vi "dfd_Calculate FIR Transposed.vi"(4 "coef idx":T1={"start"=0, "stepsize"=1}, 5 "#taps per phase":i32, 6 "coef":i64[](array[numeric]), 7 "Fwldiff":i16, 9 "state idx":T1={"start"=0, "stepsize"=1}, 10 "state in":i64[](array[numeric]), 11 "x":i64) -> (2 "state out":i64[](array[numeric]))   [LabVIEW 2017, in "NI_DigFilter_FXP.lvlib"]
uses:
  <vilib>/addons/Digital Filter Design/NI_DigFilter_FXP.lvlib
  <vilib>/addons/Digital Filter Design/_Objects.llb/dfd_Index Config.ctl
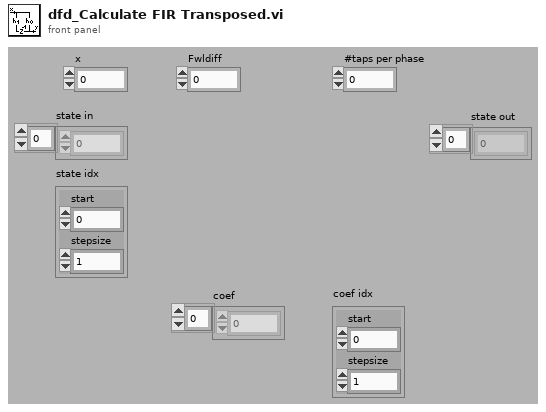
[diagram p1: front panel]
types:
  T1 = typedef "dfd_Index Config.ctl" = cluster{"start":i32, "stepsize":i32}
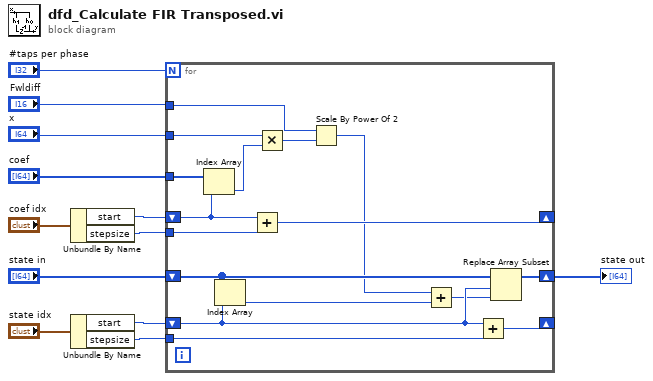
[diagram p0: block diagram]
diagram:
  n1 = Unbundle By Name("coef idx") -> ("start"=w12:i32, "stepsize"=w11:i32)
  n2 = Unbundle By Name("state idx") -> ("start"=w9:i32, "stepsize"=w10:i32)
  n3 = for {
    N: "#taps per phase" -> [_]
    shift-right: [w23] -> w2
    shift-left: "state in" -> [w24]
    shift-right: [w25] -> _
    shift-left: w12 -> [w27]
    tunnel: "coef" -> [w28]
    tunnel: w11 -> [w26]
    tunnel: "x" -> [w17]
    shift-right: [w20] -> _
    shift-left: w9 -> [w22]
    tunnel: w10 -> [w21]
    tunnel: "Fwldiff" -> [w13]
    n4 = Index Array(array=w28, index=w27) -> (element=w16:i64)
    n5 = Index Array(array=w24, index=w22) -> (element=w18:i64)
    n6 = Add(x=w27, y=w26) -> (x+y=w25:i32)
    n7 = Multiply(x=w17, y=w16) -> (x*y=w15:i64)
    n8 = Scale By Power Of 2(n=w13, x=w15) -> (x*2^n=w14:i64)
    n9 = Add(x=w14, y=w18) -> (x+y=w19:i64)
    n10 = Add(x=w22, y=w21) -> (x+y=w20:i32)
    n11 = Replace Array Subset(array=w24, new element=w19, index=w22) -> (w23:i64[])
  }
  "state out" <- w2
